vi "状态参数解析.vi"(8 "error in (no error)":errorcluster caption="错误输入（无错误）", 11 "字符串":string) -> (0 "error out":errorcluster caption="错误输出", 3 "簇":T1 {"门状态" items=["关闭", "打开"]; "采样模式" items=["定时留样"=1, "时间等比"=2, "同步留样"=3, "外控留样"=4, "超标留样"=5]; "工作进程" items=["清洗管路初始化", "采样瓶位置初始化", "采样瓶排空", "清洗管下降", "采样瓶清洗", "清洗管上升", "外置泵延时", "管路润洗", "进样1", "进样2", "排空管路", "采样瓶位置调整", "待机"]; "仪器时间" format="%<%Y/%m/%d %H:%M:%S>T"; "工作状态" items=["停止", "运行"]})   [LabVIEW 2016, in "超标留样集成.lvlib" / "德润DR803F超标留样.lvlib"]
panel:
  out "年":i32
  out "长度":i32
  out "时间标识":timestamp
  out "仪器时间1111":string
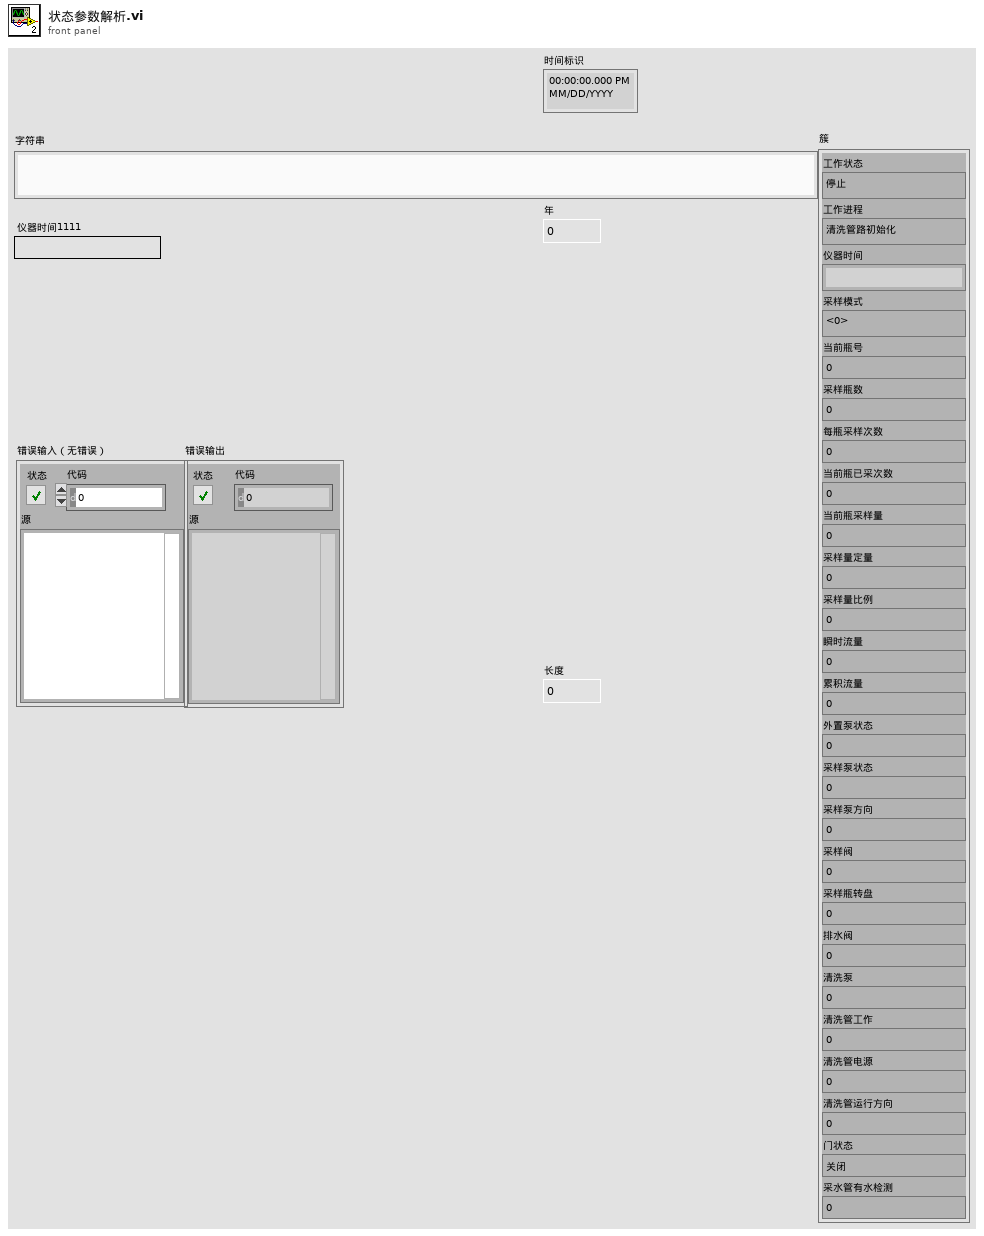
[diagram p1: front panel]
types:
  T1 = cluster{"工作状态":u16, "工作进程":u16, "仪器时间":timestamp, "采样模式":u16, "当前瓶号":dbl, "采样瓶数":dbl, "每瓶采样次数":dbl, "当前瓶已采次数":dbl, "当前瓶采样量":dbl, "采样量定量":dbl, "采样量比例":dbl, "瞬时流量":dbl, "累积流量":dbl, "外置泵状态":dbl, "采样泵状态":dbl, "采样泵方向":dbl, "采样阀":dbl, "采样瓶转盘":dbl, "排水阀":dbl, "清洗泵":dbl, "清洗管工作":dbl, "清洗管电源":dbl, "清洗管运行方向":dbl, "门状态":u16, "采水管有水检测":dbl}
  T2 = typedef "LVDateTimeRec.ctl" = cluster{"秒数的小数部分":dbl, "秒":i32, "分":i32, "时":i32, "日":i32, "月":i32, "年":i32, "天数（周）":i32, "天数（年）":i32, "DST":i32}
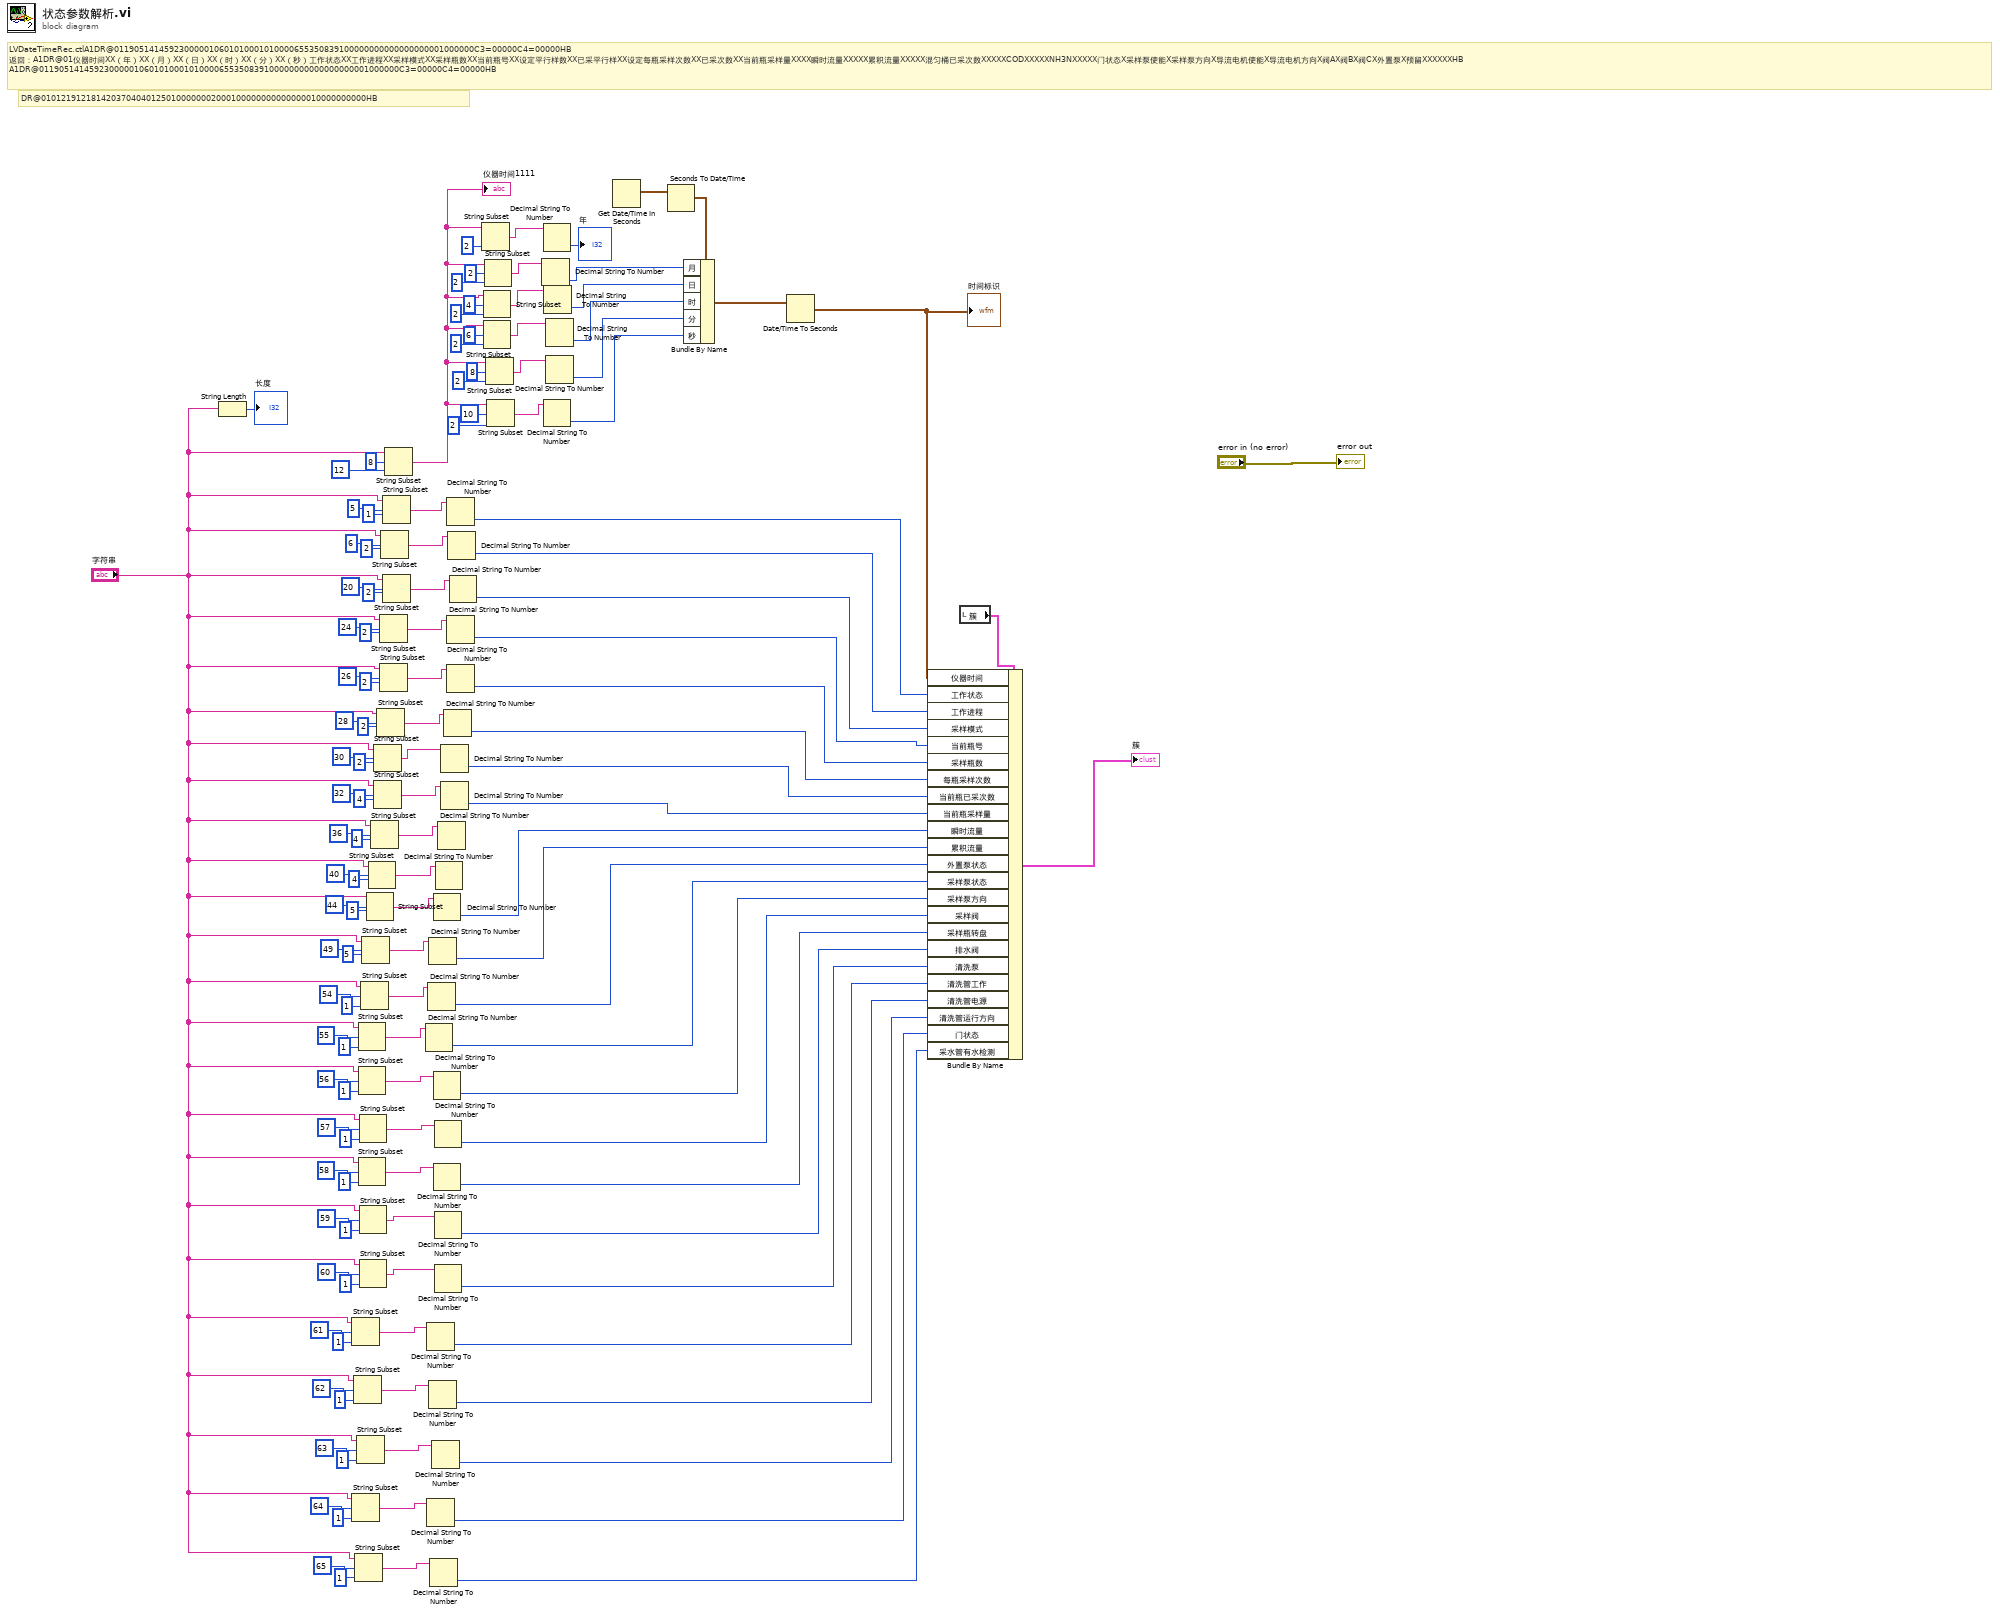
[diagram p0: block diagram]
diagram:
  # "DR@01012191218142037040401250100000002000100000000000000010000000000HB"
  # "LVDateTimeRec.ctlA1DR@011905141459230000010601010001010000655350839100000000000000000001000000C3=00000C4=00000HB\n返回：A1DR@01仪器时间XX（年）XX（月）XX（日）XX（时）XX（分）XX（秒）工作状态XX工作进程XX采样模式XX采样瓶数XX当前瓶号XX设定平行样数XX已采平行样XX设定每瓶采样次数XX已采次数XX当前瓶采样量XXXX瞬时流量XXXXX累积流量XXXXX混匀桶已采次数XXXXXCODXXXXXNH3NXXXXX门状态X采样泵使能X采样泵方向X导流电机使能X导流电机方向X阀AX阀BX阀CX外置泵X预留XXXXXXHB\nA1DR@011905141459230000010601010001010000655350839100000000000000000001000000C3=00000C4=00000HB"
  n1 = String Length(string="字符串") -> (length=→"长度":i32)
  n2 = String Subset(string="字符串", offset (0)=61 ("偏移量(0)"), length (rest)=1 ("长度（剩余）")) -> (substring=w24:string)
  n3 = String Subset(string="字符串", offset (0)=64 ("偏移量(0)"), length (rest)=1 ("长度（剩余）")) -> (substring=w11:string)
  n4 = String Subset(string="字符串", offset (0)=62 ("偏移量(0)"), length (rest)=1 ("长度（剩余）")) -> (substring=w22:string)
  n5 = String Subset(string="字符串", offset (0)=65 ("偏移量(0)"), length (rest)=1 ("长度（剩余）")) -> (substring=w16:string)
  n6 = String Subset(string="字符串", offset (0)=63 ("偏移量(0)"), length (rest)=1 ("长度（剩余）")) -> (substring=w17:string)
  n7 = String Subset(string="字符串", offset (0)=55 ("偏移量(0)"), length (rest)=1 ("长度（剩余）")) -> (substring=w45:string)
  n8 = String Subset(string="字符串", offset (0)=56 ("偏移量(0)"), length (rest)=1 ("长度（剩余）")) -> (substring=w44:string)
  n9 = String Subset(string="字符串", offset (0)=58 ("偏移量(0)"), length (rest)=1 ("长度（剩余）")) -> (substring=w35:string)
  n10 = String Subset(string="字符串", offset (0)=57 ("偏移量(0)"), length (rest)=1 ("长度（剩余）")) -> (substring=w37:string)
  n11 = String Subset(string="字符串", offset (0)=59 ("偏移量(0)"), length (rest)=1 ("长度（剩余）")) -> (substring=w27:string)
  n12 = String Subset(string="字符串", offset (0)=60 ("偏移量(0)"), length (rest)=1 ("长度（剩余）")) -> (substring=w23:string)
  n13 = String Subset(string="字符串", offset (0)=54 ("偏移量(0)"), length (rest)=1 ("长度（剩余）")) -> (substring=w51:string)
  n14 = String Subset(string="字符串", offset (0)=49 ("偏移量(0)"), length (rest)=5 ("长度（剩余）")) -> (substring=w53:string)
  n15 = String Subset(string="字符串", offset (0)=44 ("偏移量(0)"), length (rest)=5 ("长度（剩余）")) -> (substring=w59:string)
  n16 = String Subset(string="字符串", offset (0)=40 ("偏移量(0)"), length (rest)=4 ("长度（剩余）")) -> (substring=w60:string)
  n17 = String Subset(string="字符串", offset (0)=36 ("偏移量(0)"), length (rest)=4 ("长度（剩余）")) -> (substring=w67:string)
  n18 = String Subset(string="字符串", offset (0)=30 ("偏移量(0)"), length (rest)=2 ("长度（剩余）")) -> (substring=w68:string)
  n19 = String Subset(string="字符串", offset (0)=32 ("偏移量(0)"), length (rest)=4 ("长度（剩余）")) -> (substring=w69:string)
  n20 = String Subset(string="字符串", offset (0)=28 ("偏移量(0)"), length (rest)=2 ("长度（剩余）")) -> (substring=w76:string)
  n21 = String Subset(string="字符串", offset (0)=24 ("偏移量(0)"), length (rest)=2 ("长度（剩余）")) -> (substring=w84:string)
  n22 = String Subset(string="字符串", offset (0)=26 ("偏移量(0)"), length (rest)=2 ("长度（剩余）")) -> (substring=w83:string)
  n23 = String Subset(string="字符串", offset (0)=6 ("偏移量(0)"), length (rest)=2 ("长度（剩余）")) -> (substring=w91:string)
  n24 = String Subset(string="字符串", offset (0)=5 ("偏移量(0)"), length (rest)=1 ("长度（剩余）")) -> (substring=w94:string)
  n25 = String Subset(string="字符串", offset (0)=20 ("偏移量(0)"), length (rest)=2 ("长度（剩余）")) -> (substring=w90:string)
  n26 = String Subset(string="字符串", offset (0)=8 ("偏移量(0)"), length (rest)=12 ("长度（剩余）")) -> (substring=w114:string)
  "仪器时间1111" <- w114
  n27 = Decimal String To Number(string=w45) -> (number=w41:i32)  [unwired: 2 in, 1 out]
  n28 = Decimal String To Number(string=w24) -> (number=w8:i32)  [unwired: 2 in, 1 out]
  n29 = Decimal String To Number(string=w11) -> (number=w5:i32)  [unwired: 2 in, 1 out]
  n30 = Decimal String To Number(string=w51) -> (number=w48:i32)  [unwired: 2 in, 1 out]
  n31 = Decimal String To Number(string=w53) -> (number=w52:i32)  [unwired: 2 in, 1 out]
  n32 = Decimal String To Number(string=w22) -> (number=w7:i32)  [unwired: 2 in, 1 out]
  n33 = Decimal String To Number(string=w16) -> (number=w4:i32)  [unwired: 2 in, 1 out]
  n34 = Decimal String To Number(string=w17) -> (number=w6:i32)  [unwired: 2 in, 1 out]
  n35 = Decimal String To Number(string=w59) -> (number=w56:i32)  [unwired: 2 in, 1 out]
  n36 = Decimal String To Number(string=w44) -> (number=w40:i32)  [unwired: 2 in, 1 out]
  n37 = Decimal String To Number(string=w35) -> (number=w32:i32)  [unwired: 2 in, 1 out]
  n38 = Decimal String To Number(string=w37) -> (number=w36:i32)  [unwired: 2 in, 1 out]
  n39 = Decimal String To Number(string=w27) -> (number=w10:i32)  [unwired: 2 in, 1 out]
  n40 = Decimal String To Number(string=w23) -> (number=w9:i32)  [unwired: 2 in, 1 out]
  n41 = Decimal String To Number(string=w60) -> ()  [unwired: 2 in, 2 out]
  n42 = Decimal String To Number(string=w67) -> ()  [unwired: 2 in, 2 out]
  n43 = Decimal String To Number(string=w68) -> (number=w64:i32)  [unwired: 2 in, 1 out]
  n44 = Decimal String To Number(string=w69) -> (number=w63:i32)  [unwired: 2 in, 1 out]
  n45 = Decimal String To Number(string=w76) -> (number=w74:i32)  [unwired: 2 in, 1 out]
  n46 = Decimal String To Number(string=w94) -> (number=w93:i32)  [unwired: 2 in, 1 out]
  n47 = Decimal String To Number(string=w84) -> (number=w80:i32)  [unwired: 2 in, 1 out]
  n48 = Decimal String To Number(string=w83) -> (number=w79:i32)  [unwired: 2 in, 1 out]
  n49 = Decimal String To Number(string=w91) -> (number=w92:i32)  [unwired: 2 in, 1 out]
  n50 = Decimal String To Number(string=w90) -> (number=w87:i32)  [unwired: 2 in, 1 out]
  n51 = String Subset(string=w114, length (rest)=2 ("长度（剩余）")) -> (substring=w101:string)  [unwired: 1 in]
  n52 = String Subset(string=w114, offset (0)=4 ("偏移量(0)"), length (rest)=2 ("长度（剩余）")) -> (substring=w118:string)
  n53 = String Subset(string=w114, offset (0)=6 ("偏移量(0)"), length (rest)=2 ("长度（剩余）")) -> (substring=w107:string)
  n54 = String Subset(string=w114, offset (0)=2 ("偏移量(0)"), length (rest)=2 ("长度（剩余）")) -> (substring=w122:string)
  n55 = String Subset(string=w114, offset (0)=8 ("偏移量(0)"), length (rest)=2 ("长度（剩余）")) -> (substring=w108:string)
  n56 = String Subset(string=w114, offset (0)=10 ("偏移量(0)"), length (rest)=2 ("长度（剩余）")) -> (substring=w109:string)
  n57 = Decimal String To Number(string=w122) -> (number=w121:i32)  [unwired: 2 in, 1 out]
  n58 = Decimal String To Number(string=w101) -> (number=→"年":i32)  [unwired: 2 in, 1 out]
  n59 = Decimal String To Number(string=w109) -> (number=w104:i32)  [unwired: 2 in, 1 out]
  n60 = Decimal String To Number(string=w118) -> (number=w117:i32)  [unwired: 2 in, 1 out]
  n61 = Decimal String To Number(string=w107) -> (number=w106:i32)  [unwired: 2 in, 1 out]
  n62 = Decimal String To Number(string=w108) -> (number=w105:i32)  [unwired: 2 in, 1 out]
  n63 = Get Date/Time In Seconds() -> (seconds since 1Jan1904=w103:timestamp)
  n64 = Seconds To Date/Time(time stamp (now)=w103) -> (date time rec=w102:T2)  [unwired: 1 in]
  n65 = Bundle By Name(cluster=w102, "月"=w121, "日"=w117, "时"=w106, "分"=w105, "秒"=w104) -> (w126:T2)
  n66 = Date/Time To Seconds(2:w126) -> (0:w99:timestamp)  [unwired: 1 in]
  "时间标识" <- w99
  n67 = local read "簇"() -> (w75:T1)
  n68 = Bundle By Name(cluster=w75, "仪器时间"=w99, "工作状态"=w93, "工作进程"=w92, "采样模式"=w87, "当前瓶号"=w80, "采样瓶数"=w79, "每瓶采样次数"=w74, "当前瓶已采次数"=w64, "当前瓶采样量"=w63, "瞬时流量"=w56, "累积流量"=w52, "外置泵状态"=w48, "采样泵状态"=w41, "采样泵方向"=w40, "采样阀"=w36, "采样瓶转盘"=w32, "排水阀"=w10, "清洗泵"=w9, "清洗管工作"=w8, "清洗管电源"=w7, "清洗管运行方向"=w6, "门状态"=w5, "采水管有水检测"=w4) -> (→"簇":T1)
  "error out" <- "error in (no error)"
